vi "FTW-Container-Support-XML-SerializeNode.vi"(0 "XML Node":refnum<k20>, 5 "Indent Characters":string, 7 "Indent Level":i32=1, 11 "error in":errorcluster) -> (4 "XML Node out":refnum<k20>, 6 "Serialized Node":string, 15 "error out":errorcluster)   [LabVIEW 2015, in "FTW-Container.lvclass"]
uses:
  FTW-Container.lvclass
  JSON/FTW-JSON-CompositeType.ctl
  JSON/FTW-JSON-Escape.vi
  Error/FTW-ERR-ThrowError.vi
panel:
  # "Inputs"
  # "Outputs"
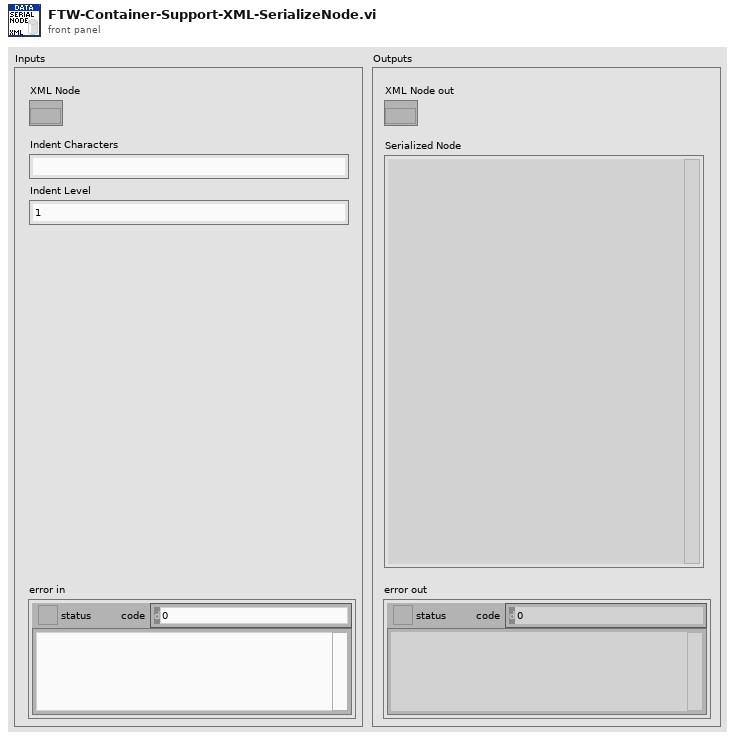
[diagram p1: front panel]
types:
  T1 = typedef "FTW-JSON-CompositeType.ctl" = enum16{"Object", "Array"}
  T2 = typedef "FTW-JSON-Datatype.ctl" = enum16{"Object", "Array", "String", "Number", "Boolean", "NULL", "<Refnum>", "<Enum>", "<Unknown>"}
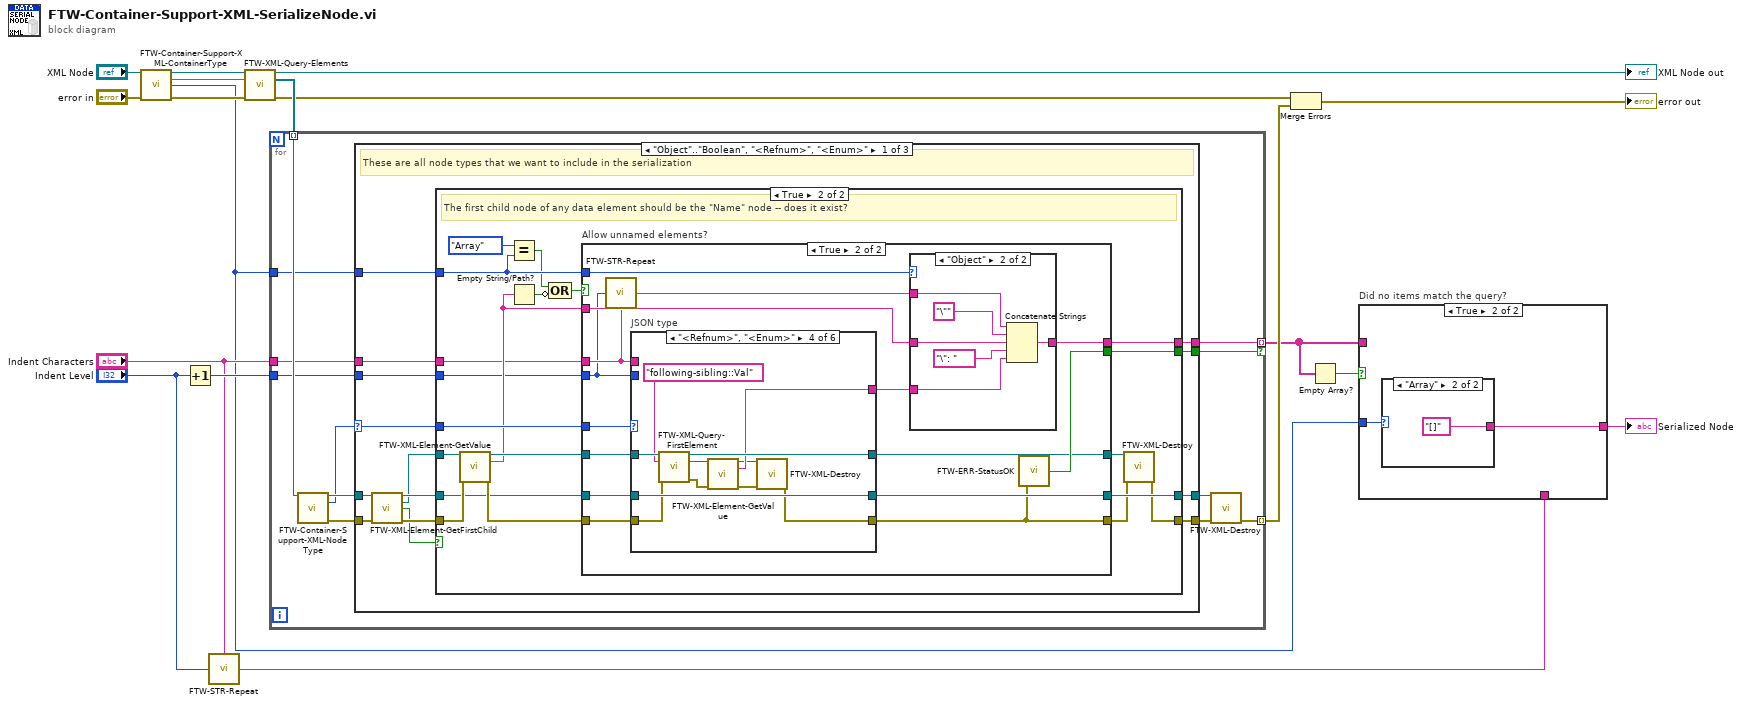
[diagram p0: block diagram]
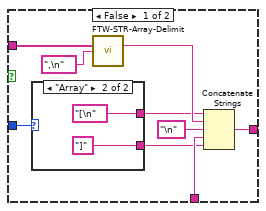
[diagram p2: hidden frame]
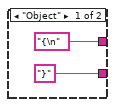
[diagram p3: hidden frame]
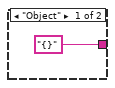
[diagram p4: hidden frame]
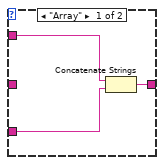
[diagram p7: hidden frame]
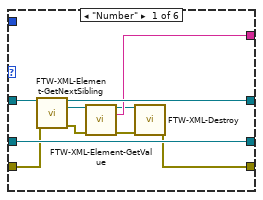
[diagram p8: hidden frame]
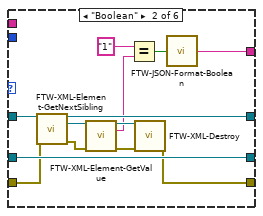
[diagram p9: hidden frame]
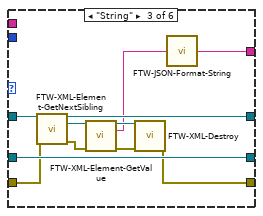
[diagram p10: hidden frame]
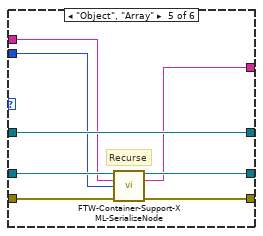
[diagram p11: hidden frame]
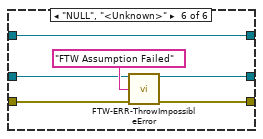
[diagram p12: hidden frame]
diagram:
  n1 = call "FTW-Container-Support-XML-ContainerType.vi"("Element Node"="XML Node", "error in"="error in") -> ("Element Node out"=w6:refnum<k20>, "Parent XPath Query"=w4:string, "Parent Type"=w3:T1, "error out"=w5:errorcluster)  [unwired: 9 in, 1 out]
  n2 = Increment(x="Indent Level") -> (x+1=w9:i32)
  n3 = call "FTW-STR-Repeat.vi"("Times to Repeat"="Indent Level", "String to Repeat"="Indent Characters") -> ("Indented String"=w11:string)
  n4 = call "FTW-XML-Query-Elements.vi"("XML Node"=w6, "XPath Query"=w4, "error in"=w5) -> ("XML Node out"=→"XML Node out":refnum<k20>, "Matching Nodes"=w18:refnum<k20>[], "error out"=w16:errorcluster)  [unwired: 9 in, 1 out]
  n5 = for {
    tunnel: w18 -> [w30] mode=indexing
    tunnel: [w27] -> w13 mode=indexing if=w23
    tunnel: [w26] -> w17 mode=indexing
    tunnel: "Indent Characters" -> [w22]
    tunnel: w9 -> [w21]
    tunnel: w3 -> [w20]
    n6 = call "FTW-Container-Support-XML-NodeType.vi"("Element Node"=w30) -> ("Element Node out"=w29:refnum<k20>, "JSON Type"=w24:T2, "error out"=w28:errorcluster)  [unwired: 11 in, 1 out]
    n7 = case shown="\"Object\"..\"Boolean\", \"<Refnum>\", \"<Enum>\"" w24 {
      selector: w24 -> [w36 _ _]
      tunnel: w28 -> [w31 w152 w155]
      tunnel: [w37 w152 w155] -> w25
      tunnel: w29 -> [w32 w153 w154]
      tunnel: [w39 _ _] -> w27
      tunnel: [w40 w153 w154] -> w19
      tunnel: [w38 _ _] -> w23
      tunnel: w22 -> [w35 _ _]
      tunnel: w21 -> [w34 _ _]
      tunnel: w20 -> [w33 _ _]
      frame "Object".."Boolean", "<Refnum>", "<Enum>" {
        # "These are all node types that we want to include in the serialization"
        n8 = call "FTW-XML-Element-GetFirstChild.vi"("Element Node"=w32, "error in"=w31) -> ("Element Node out"=w42:refnum<k20>, "First Child Element Node"=w41:refnum<k20>, "Found?"=w43:bool, "error out"=w44:errorcluster)  [unwired: 10 in]
        n9 = case shown="True" w43 {
          tunnel: w42 -> [w45 w61]
          tunnel: w44 -> [w46 w66]
          tunnel: w36 -> [_ w60]
          tunnel: w41 -> [_ w65]
          tunnel: [w45 w64] -> w40
          tunnel: [w46 w55] -> w37
          tunnel: [_ w59] -> w39
          tunnel: [_ w51] -> w38
          tunnel: w35 -> [_ w57]
          tunnel: w34 -> [_ w56]
          tunnel: w33 -> [_ w50]
          frame False {
            # "A child node did not exist; therefore it does not need to be destroyed"
          }
          frame True {
            # "The first child node of any data element should be the \"Name\" node -- does it exist?"
            n10 = call "FTW-XML-Element-GetValue.vi"("XML Node"=w65, "error in"=w66) -> ("XML Node out"=w62:refnum<k20>, "Node Text Value"=w58:string, "error out"=w63:errorcluster)  [unwired: 11 in]
            n11 = Equal?(x=FTW-JSON-CompositeType."Array", y=w50) -> (x = y?=w49:bool)
            n12 = Empty String/Path?(string/path=w58) -> (empty?=w48:bool)
            n13 = Compound Arithmetic op=OR(w49, invert w48) -> (w52:bool)
            n14 = case "Allow unnamed elements?" shown="True" w52 {
              tunnel: [w67 w76] -> w64
              tunnel: w63 -> [w69 w84]
              tunnel: w62 -> [w68 w83]
              tunnel: w61 -> [w67 w82]
              tunnel: w60 -> [_ w81]
              tunnel: [w69 w75] -> w54
              tunnel: [_ w80] -> w59
              tunnel: w58 -> [_ w79]
              tunnel: w50 -> [_ w78]
              tunnel: w57 -> [_ w71]
              tunnel: w56 -> [_ w70]
              tunnel: [w68 w73] -> w53
              tunnel: [_ w74] -> w51
              frame False {
              }
              frame True {
                n15 = call "FTW-STR-Repeat.vi"("Times to Repeat"=w70, "String to Repeat"=w71) -> ("Indented String"=w72:string)
                n16 = case "JSON type" shown="\"<Refnum>\", \"<Enum>\"" w81 {
                  tunnel: [w94 w108 w119 w129 w143 w151] -> w75
                  tunnel: w82 -> [w98 w112 w123 w133 w145 w147]
                  tunnel: [w98 w112 w123 w133 w142 w147] -> w76
                  tunnel: w83 -> [w102 w115 w126 w137 w146 w149]
                  tunnel: w84 -> [w97 w111 w122 w132 w144 w148]
                  tunnel: [w103 w116 w127 w138 w146 w149] -> w73
                  tunnel: [w100 w104 w117 w135 w140 _] -> w77
                  tunnel: w71 -> [_ _ _ _ w141 _]
                  tunnel: w70 -> [_ _ _ _ w139 _]
                  frame "Number" {
                    n17 = call "FTW-XML-Element-GetNextSibling.vi"("XML Node"=w102, "error in"=w97) -> ("XML Node out"=w103:refnum<k20>, "Next Sibling"=w101:refnum<k20>, "error out"=w99:errorcluster)  [unwired: 10 in, 1 out]
                    n18 = call "FTW-XML-Element-GetValue.vi"("XML Node"=w101, "error in"=w99) -> ("XML Node out"=w96:refnum<k20>, "Node Text Value"=w100:string, "error out"=w95:errorcluster)  [unwired: 11 in]
                    n19 = call "FTW-XML-Destroy.vi"("XML Node"=w96, "error in"=w95) -> ("error out"=w94:errorcluster)  [unwired: 13 in]
                  }
                  frame "Boolean" {
                    n20 = call "FTW-XML-Element-GetNextSibling.vi"("XML Node"=w115, "error in"=w111) -> ("XML Node out"=w116:refnum<k20>, "Next Sibling"=w114:refnum<k20>, "error out"=w113:errorcluster)  [unwired: 10 in, 1 out]
                    n21 = call "FTW-XML-Element-GetValue.vi"("XML Node"=w114, "error in"=w113) -> ("XML Node out"=w110:refnum<k20>, "Node Text Value"=w105:string, "error out"=w109:errorcluster)  [unwired: 11 in]
                    n22 = Equal?(x="1", y=w105) -> (x = y?=w107:bool)
                    n23 = call "FTW-XML-Destroy.vi"("XML Node"=w110, "error in"=w109) -> ("error out"=w108:errorcluster)  [unwired: 13 in]
                    n24 = call "FTW-JSON-Format-Boolean.vi"("LabVIEW Boolean"=w107) -> ("JSON Boolean"=w104:string)
                  }
                  frame "String" {
                    n25 = call "FTW-XML-Element-GetNextSibling.vi"("XML Node"=w126, "error in"=w122) -> ("XML Node out"=w127:refnum<k20>, "Next Sibling"=w125:refnum<k20>, "error out"=w124:errorcluster)  [unwired: 10 in, 1 out]
                    n26 = call "FTW-XML-Element-GetValue.vi"("XML Node"=w125, "error in"=w124) -> ("XML Node out"=w121:refnum<k20>, "Node Text Value"=w118:string, "error out"=w120:errorcluster)  [unwired: 11 in]
                    n27 = call "FTW-XML-Destroy.vi"("XML Node"=w121, "error in"=w120) -> ("error out"=w119:errorcluster)  [unwired: 13 in]
                    n28 = call "FTW-JSON-Format-String.vi"("LabVIEW String"=w118) -> ("JSON String"=w117:string)
                  }
                  frame "<Refnum>", "<Enum>" {
                    n29 = call "FTW-XML-Query-FirstElement.vi"("XML Node"=w137, "XPath Query"="following-sibling::Val", "error in"=w132) -> ("XML Node out"=w138:refnum<k20>, "First Matched Element"=w136:refnum<k20>, "error out"=w134:errorcluster)  [unwired: 8 in, 2 out]
                    n30 = call "FTW-XML-Element-GetValue.vi"("XML Node"=w136, "error in"=w134) -> ("XML Node out"=w131:refnum<k20>, "Node Text Value"=w135:string, "error out"=w130:errorcluster)  [unwired: 11 in]
                    n31 = call "FTW-XML-Destroy.vi"("XML Node"=w131, "error in"=w130) -> ("error out"=w129:errorcluster)  [unwired: 13 in]
                  }
                  frame "Object", "Array" {
                    # "Recurse"
                    n32 = call "FTW-Container-Support-XML-SerializeNode.vi"("XML Node"=w145, "Indent Characters"=w141, "Indent Level"=w139, "error in"=w144) -> ("XML Node out"=w142:refnum<k20>, "Serialized Node"=w140:string, "error out"=w143:errorcluster)  [unwired: 9 in]
                  }
                  frame "NULL", "<Unknown>" {
                    n33 = call "FTW-ERR-ThrowImpossibleError.vi"("Reason this error should never happen"="FTW Assumption Failed", "error in"=w148) -> ("error out"=w151:errorcluster)  [unwired: 13 in]
                  }
                }
                n34 = case shown="\"Object\"" w78 {
                  tunnel: w72 -> [w87 w93]
                  tunnel: w79 -> [_ w92]
                  tunnel: [w86 w90] -> w80
                  tunnel: w77 -> [w85 w89]
                  frame "Array" {
                    n35 = Concatenate Strings(w87, w85) -> (w86:string)
                  }
                  frame "Object" {
                    n36 = Concatenate Strings(w93, "\"" ("String to Repeat"), w92, "\": " ("String to Repeat"), w89) -> (w90:string)
                  }
                }
                n37 = call "FTW-ERR-StatusOK.vi"("error to check"=w75) -> ("Status OK?"=w74:bool)
              }
            }
            n38 = call "FTW-XML-Destroy.vi"("XML Node"=w53, "error in"=w54) -> ("error out"=w55:errorcluster)  [unwired: 13 in]
          }
        }
      }
      frame "NULL" {
        # "There is no mapping from LV to the JSON null type, therefore, we never expect this case."
      }
      frame "<Unknown>" {
        # "This case is most likely a node type in the LabVIEW Schema that is unnecessary to parse."
      }
    }
    n39 = call "FTW-XML-Destroy.vi"("XML Node"=w19, "error in"=w25) -> ("error out"=w26:errorcluster)  [unwired: 13 in]
  }
  n40 = Merge Errors(w16, w17) -> (→"error out":errorcluster)
  n41 = Empty Array?(array=w13) -> (empty?=w12:bool)
  n42 = case "Did no items match the query?" shown="True" w12 {
    tunnel: [w161 w169] -> w14
    tunnel: w13 -> [w160 _]
    tunnel: w11 -> [w159 _]
    tunnel: w3 -> [w156 w170]
    frame False {
      n43 = case shown="\"Array\"" w156 {
        tunnel: ["{\n" ("String to Repeat") "[\n" ("String to Repeat")] -> w158
        tunnel: ["}" ("String to Repeat") "]" ("String to Repeat")] -> w157
        frame "Object" {
        }
        frame "Array" {
        }
      }
      n44 = call "FTW-STR-Array-Delimit.vi"("Array of Strings"=w160, "Delimiter"=",\n" ("String to Repeat")) -> ("Delimited String"=w163:string)  [unwired: 13 in]
      n45 = Concatenate Strings(w158, w163, "\n" ("String to Repeat"), w159, w157) -> (w161:string)
    }
    frame True {
      n46 = case shown="\"Array\"" w170 {
        tunnel: ["{}" ("String to Repeat") "[]" ("String to Repeat")] -> w169
        frame "Object" {
        }
        frame "Array" {
        }
      }
    }
  }
  "Serialized Node" <- w14
